vi "guess_config_file_name.vi"() -> (0 "config file path":path)   [LabVIEW 2010]
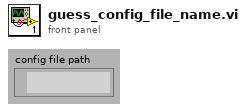
[diagram p1: front panel]
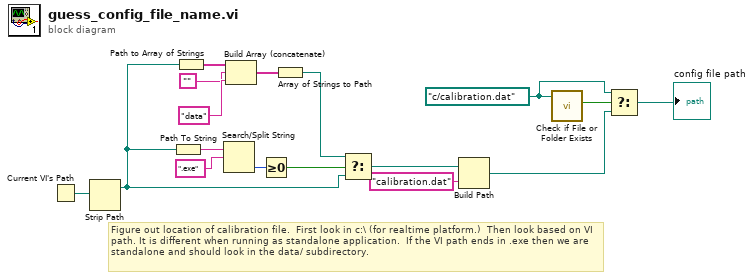
[diagram p0: block diagram]
diagram:
  w3 = path "c:/calibration.dat" ("path")
  # "Figure out location of calibration file.  First look in c:\\ (for realtime platform.)  Then look based on VI path. It is different when running as standalone application.  If the VI path ends in .exe then we are standalone and should look in the data/ subdirectory."
  n1 = Current VI's Path() -> (path=w6:path)
  n2 = Strip Path(path=w6) -> (stripped path=w15:path)  [unwired: 1 out]
  n3 = Path To String(path=w15) -> (string=w11:string)
  n4 = Path to Array of Strings(0:w15) -> (2:w7:string[])  [unwired: 1 out]
  n5 = Search/Split String(string=w11, search string/char (-)=".exe" ("regular expression")) -> (offset of match=w12:i32)  [unwired: 3 out]
  n6 = Build Array (concatenate)(w7, "", "data") -> (w9:string[])
  n7 = Greater Or Equal To 0?(x=w12) -> (x >= 0?=w13:bool)
  n8 = Array of Strings to Path(0:w9) -> (2:w14:path)  [unwired: 1 out]
  n9 = Select(t=w14, s=w13, f=w15) -> (s? t:f=w16:path)
  n10 = Build Path(base path=w16, name or relative path="calibration.dat") -> (appended path=w1:path)
  n11 = call <vilib>:"Check if File or Folder Exists.vi"("path"=w3) -> ("file or folder exists?"=w4:bool)  [unwired: 1 in, 9 out]
  n12 = Select(t=w3, s=w4, f=w1) -> (s? t:f=→"config file path":path)
